vi "Plugins Folder Config.vi"(8 "error in (no error)":errorcluster, 11 "GUI Manager Module in":refnum<class "GUI Manager Module.lvclass">) -> (0 "error out":errorcluster, 3 "GUI Manager Module out":refnum<class "GUI Manager Module.lvclass">)   [LabVIEW 2020, in "VolatusGUI.lvlib" / "GUI Manager Module.lvclass"]
uses:
  GUI Manager Module.lvclass
  C:/dev/lv20CE/relink/lv-volatus/Volatus/Module/Module.lvclass
  Volatus/Module/Module.lvclass/Module.ctl
  VolatusConfig/VolatusConfigElement/VolatusConfigElement.lvclass/VolatusConfigElement.ctl
  GUI Manager Module.lvclass/GUI Manager Module.ctl
  Volatus/Module/Config.vi
  VolatusConfig/VolatusConfigElement/Lookup Child by Name.vi
  VolatusConfig/VolatusConfigElement/Element.vi
  lv-cdm/CDM-Config/Config Element/Lookup Child by Name.vi
  Volatus/Module/Module.lvclass
  lv-cdm/CDM-Config/Config Element/Config Element.lvclass
  Volatus/VolatusAPI/VolatusAPI.lvclass
  C:/dev/lv20CE/relink/lv-volatus/VolatusGUI/GUI Manager Module/GUI Manager Module.lvclass
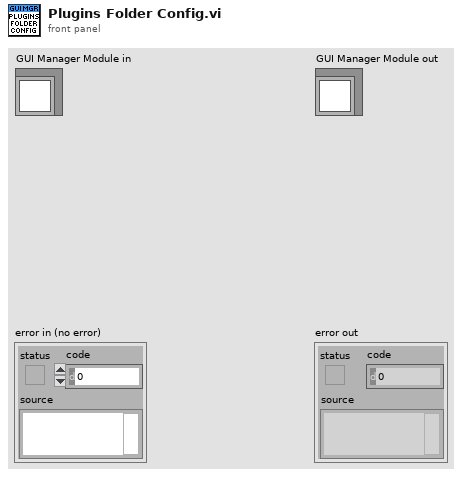
[diagram p1: front panel]
types:
  T1 = typedef "CDM-Config.lvlib/Value Type.ctl" = enum16{"String", "Number", "Bool", "Object", "Array"}
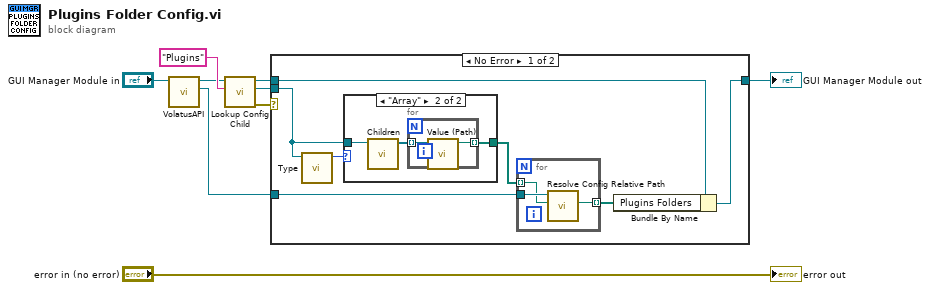
[diagram p0: block diagram]
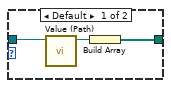
[diagram p2: hidden frame]
diagram:
  n1 = call "VolatusAPI.vi"("Module in"="GUI Manager Module in") -> ("VolatusAPI"=w6:refnum<class "VolatusAPI.lvclass">, "Module out"=w7:refnum<class "GUI Manager Module.lvclass">)  [unwired: 9 in]
  n2 = call "Lookup Config Child.vi"("Name"="Plugins", "Module in"=w7) -> ("error out"=w4:errorcluster, "Config Child"=w5:refnum<class "Config Element.lvclass">, "Module in"=w3:refnum<class "GUI Manager Module.lvclass">)  [unwired: 6 in, 1 out]
  n3 = case shown="No Error" w4 {
    tunnel: w6 -> [w13 _]
    tunnel: w5 -> [w15 _]
    tunnel: w3 -> [w12 w28]
    tunnel: [w10 w28] -> w1
    frame No Error {
      n4 = call "Type.vi"("Config Element in"=w15) -> ("Value Type"=w16:T1)  [unwired: 9 in, 1 out]
      n5 = case shown="\"Array\"" w16 {
        tunnel: w15 -> [w22 w25]
        tunnel: [w20 w23] -> w14
        frame Default {
          n6 = call "Value (Path).vi"("Config Element in"=w22) -> ("Path Value"=w21:path)  [unwired: 9 in, 1 out]
          n7 = Build Array(w21) -> (w20:path[])
        }
        frame "Array" {
          n8 = call "Children.vi"("Config Element in"=w25) -> ("Elements"=w24:refnum<class "Config Element.lvclass">[])  [unwired: 9 in, 1 out]
          n9 = for {
            tunnel: w24 -> [w27] mode=indexing
            tunnel: [w26] -> w23 mode=indexing
            n10 = call "Value (Path).vi"("Config Element in"=w27) -> ("Path Value"=w26:path)  [unwired: 9 in, 1 out]
          }
        }
      }
      n11 = for {
        tunnel: w14 -> [w18] mode=indexing
        tunnel: w13 -> [w19]
        tunnel: [w17] -> w11 mode=indexing
        n12 = call "Resolve Config Relative Path.vi"("Path"=w18, "VolatusAPI in"=w19) -> ("Resolved Path"=w17:path)  [unwired: 7 in, 2 out]
      }
      n13 = Bundle By Name(cluster=w12, "Plugins Folders"=w11) -> (w10:refnum<class "GUI Manager Module.lvclass">)
    }
    frame Error {
      # "Optional configuration"
    }
  }
  "GUI Manager Module out" <- w1
  "error out" <- "error in (no error)"
